vi "Save Workspace.vi"(8 "error in (no error)":errorcluster, 11 "Cfg Grandmaster in":refnum<class "Cfg Grandmaster.lvclass">) -> (0 "error out":errorcluster, 3 "Cfg Grandmaster out":refnum<class "Cfg Grandmaster.lvclass">)   [LabVIEW 2018, in "Configuration Grandmaster.lvlib" / "Cfg Grandmaster.lvclass"]
uses:
  Cfg Grandmaster.lvclass
  Common/Controls/Chassis Cfg Assoc.ctl
  Common/Controls/Workspace.ctl
  Common/Controls/TCP Ports.ctl
  Cfg Grandmaster.lvclass/Cfg Grandmaster.ctl
  Class Chassis BOM/Chassis BOM.lvclass/Chassis BOM.ctl
  Class Chassis BOM/Read Chassis Alias.vi
  Class Chassis BOM/Read CfgFile.vi
  Class Chassis BOM/Chassis BOM.lvclass
  <vilib>/NI/GXML/GXML.lvlib
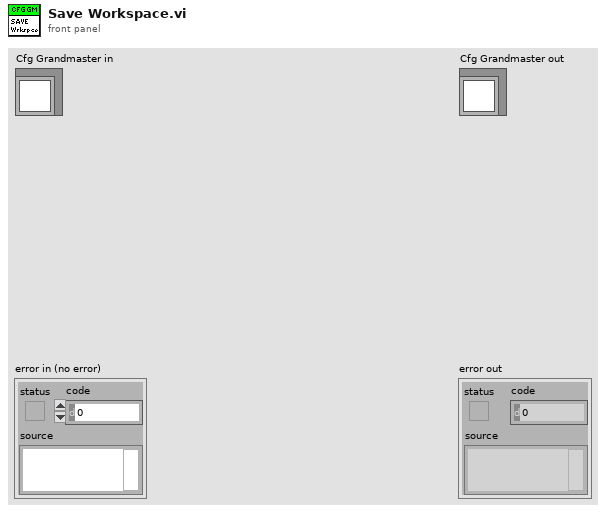
[diagram p1: front panel]
types:
  T1 = typedef "Workspace.ctl" = cluster{"Ports":T2, "GlblConfig":T3[]}
  T2 = typedef "TCP Ports.ctl" = cluster{"Port Rdr":u16, "Port HS":u16, "Port LS":u16}
  T3 = typedef "Chassis Cfg Assoc.ctl" = cluster{"Chassis Name":string, "CfgFile":path}
  T4 = typedef "ge_Cfg wChassis.ctl" = cluster{"Chassis BOM":refnum<class "Chassis BOM.lvclass">, "Chassis Cfg":refnum<class "ChassisCfg.lvclass">, "Chassis Tasks":refnum<class "Chassis Tasks.lvclass">, "HW Error":bool, "Unsvd Chgs?":bool}
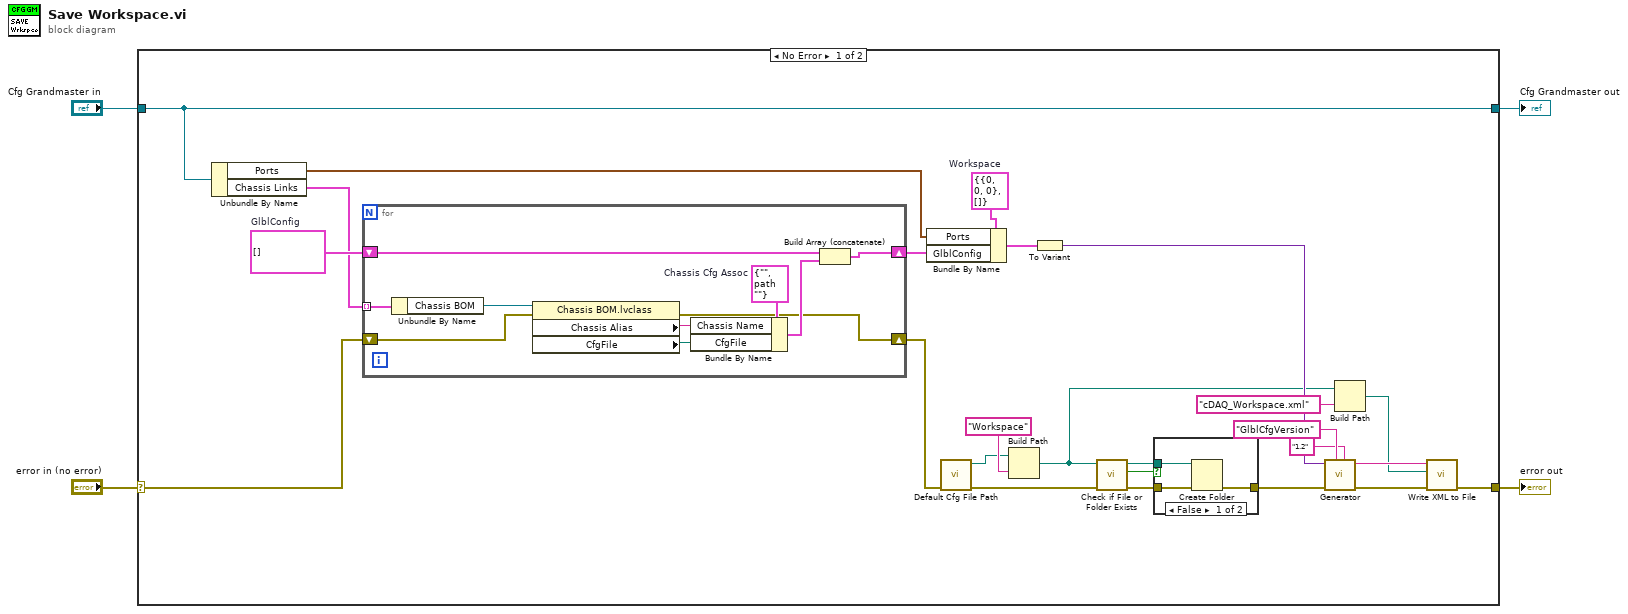
[diagram p0: block diagram]
diagram:
  n1 = case shown="No Error" "error in (no error)" {
    selector: "error in (no error)" -> [w8 w45]
    tunnel: [w9 w45] -> w3
    tunnel: [w7 w44] -> w1
    tunnel: "Cfg Grandmaster in" -> [w7 w44]
    frame No Error {
      w14 = T1 {"Ports"={"Port Rdr"=0, "Port HS"=0, "Port LS"=0}, "GlblConfig"=[]}  # Workspace
      w18 = T3[] []  # GlblConfig
      n2 = Unbundle By Name(w7) -> ("Ports"=w6:T2, "Chassis Links"=w5:T4[])
      n3 = for {
        tunnel: w5 -> [w43] mode=indexing
        shift-right: [w39] -> w13
        shift-left: w18 -> [w41]
        shift-right: [w34] -> w10
        shift-left: w8 -> [w35]
        w42 = T3 {"Chassis Name"="", "CfgFile"=path ""}  # Chassis Cfg Assoc
        n4 = Unbundle By Name(w43) -> ("Chassis BOM"=w36:refnum<class "Chassis BOM.lvclass">)
        n5 = property class="Chassis BOM.lvclass"(reference=w36, error in=w35) -> (error out=w34:errorcluster, "Chassis Alias"=w38:string, "CfgFile"=w37:path)  [unwired: 1 out]
        n6 = Bundle By Name(cluster=w42, "Chassis Name"=w38, "CfgFile"=w37) -> (w40:T3)
        n7 = Build Array (concatenate)(w41, w40) -> (w39:T3[])
      }
      n8 = Bundle By Name(cluster=w14, "Ports"=w6, "GlblConfig"=w13) -> (w12:T1)
      n9 = call "Default Cfg File Path.vi"("error in (no error)"=w10) -> ("error out"=w11:errorcluster, "Default Path"=w16:path)  [unwired: 9 in]
      n10 = Build Path(base path=w16, name or relative path="Workspace") -> (appended path=w17:path)
      n11 = To Variant(anything=w12) -> (Variant=w28:variant)
      n12 = call <vilib>:"Check if File or Folder Exists.vi"("error in (no error)"=w11, "path"=w17) -> ("error out"=w22:errorcluster, "file or folder exists?"=w23:bool, "dup path"=w24:path)  [unwired: 7 in]
      n13 = case shown="False" w23 {
        tunnel: w24 -> [w32 _]
        tunnel: w22 -> [w31 w33]
        tunnel: [w30 w33] -> w21
        frame False {
          n14 = Create Folder(path (use dialog)=w32, error in=w31) -> (error out=w30:errorcluster)  [unwired: 1 in, 2 out]
        }
        frame True {
        }
      }
      n15 = call <vilib>:"Generator.vi"("Version String"="1.2", "Version Tag Name"="GlblCfgVersion", "error in"=w21, "Variant"=w28) -> ("error out"=w29:errorcluster, "XML String Out"=w27:string)  [unwired: 6 in]
      n16 = Build Path(base path=w17, name or relative path="cDAQ_Workspace.xml") -> (appended path=w19:path)
      n17 = call <vilib>:"Write XML to File.vi"("error in"=w29, "XML File Path"=w19, "XML Input"=w27) -> ("error out"=w9:errorcluster)  [unwired: 8 in]
    }
    frame Error {
    }
  }
  "error out" <- w3
  "Cfg Grandmaster out" <- w1
